vi "skip_squid.vi"   [LabVIEW 2015]
uses:
  Global.vi
panel:
  # "Skip to next squid."
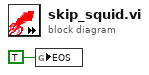
[diagram p0: block diagram]
diagram:
  n1 = global write "Global.vi" "EOS"(TRUE ("EOS")) -> ()
